vi "Teleop.vi"(10 "Match Info":T1={"Autonomous Elapsed Seconds"=0.0, "TeleOp Elapsed Seconds"=0.0, "Disabled Elapsed Seconds"=0.0, "Visited Autonomous"=FALSE, "Visited TeleOp"=FALSE, "Visited Disabled"=FALSE, "Autonomous Settings"={"Autonomous Style"=enum."Independent", "VI Refnum"=refnum}}, 11 "Call Context":T2) -> ()   [LabVIEW 2018]
doc: "This VI is called for each enabled TeleOp packet received from the DS. It is typically used to read from joysticks and other inputs and update I/O or setpoints for timed control loops. It should complete and return within 20 milliseconds or risk missing DS packets."
uses:
  <vilib>/Rock Robotics/WPI/DriverStation/WPI_DriverStationDerivedRobotMode.ctl
  <vilib>/Rock Robotics/WPI/DriverStation/WPI_DriverStationMatch Info.ctl
  <vilib>/Rock Robotics/WPI/Solenoid/WPI_SolenoidValue.ctl
  Framework/Robot Global Data.vi
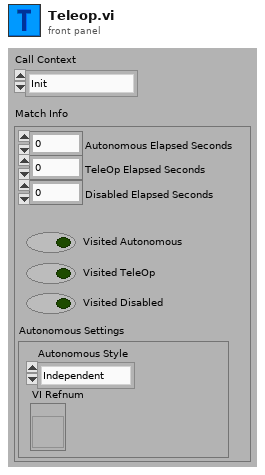
[diagram p1: front panel]
types:
  T1 = typedef "WPI_DriverStationMatch Info.ctl" = cluster{"Autonomous Elapsed Seconds":dbl, "TeleOp Elapsed Seconds":dbl, "Disabled Elapsed Seconds":dbl, "Visited Autonomous":bool, "Visited TeleOp":bool, "Visited Disabled":bool, "Autonomous Settings":cluster{"Autonomous Style":enum16{"Iterative", "Independent"}, "VI Refnum":refnum<vi>}}
  T2 = typedef "WPI_DriverStationDerivedRobotMode.ctl" = enum16{"Init", "Execute", "Stop"}
  T3 = typedef "Command Status Info.ctl" = cluster{"Name":string, "Status":T4, "notifier out":T5}
  T4 = typedef "Completion Status.ctl" = enum16{"Successful", "Aborted", "Incomplete"}
  T5 = typedef "Completion Notifier.ctl" = refnum<notifier>
  T6 = typedef "WPI_SolenoidValue.ctl" = enum16{"Off", "On", "Forward", "Reverse"}
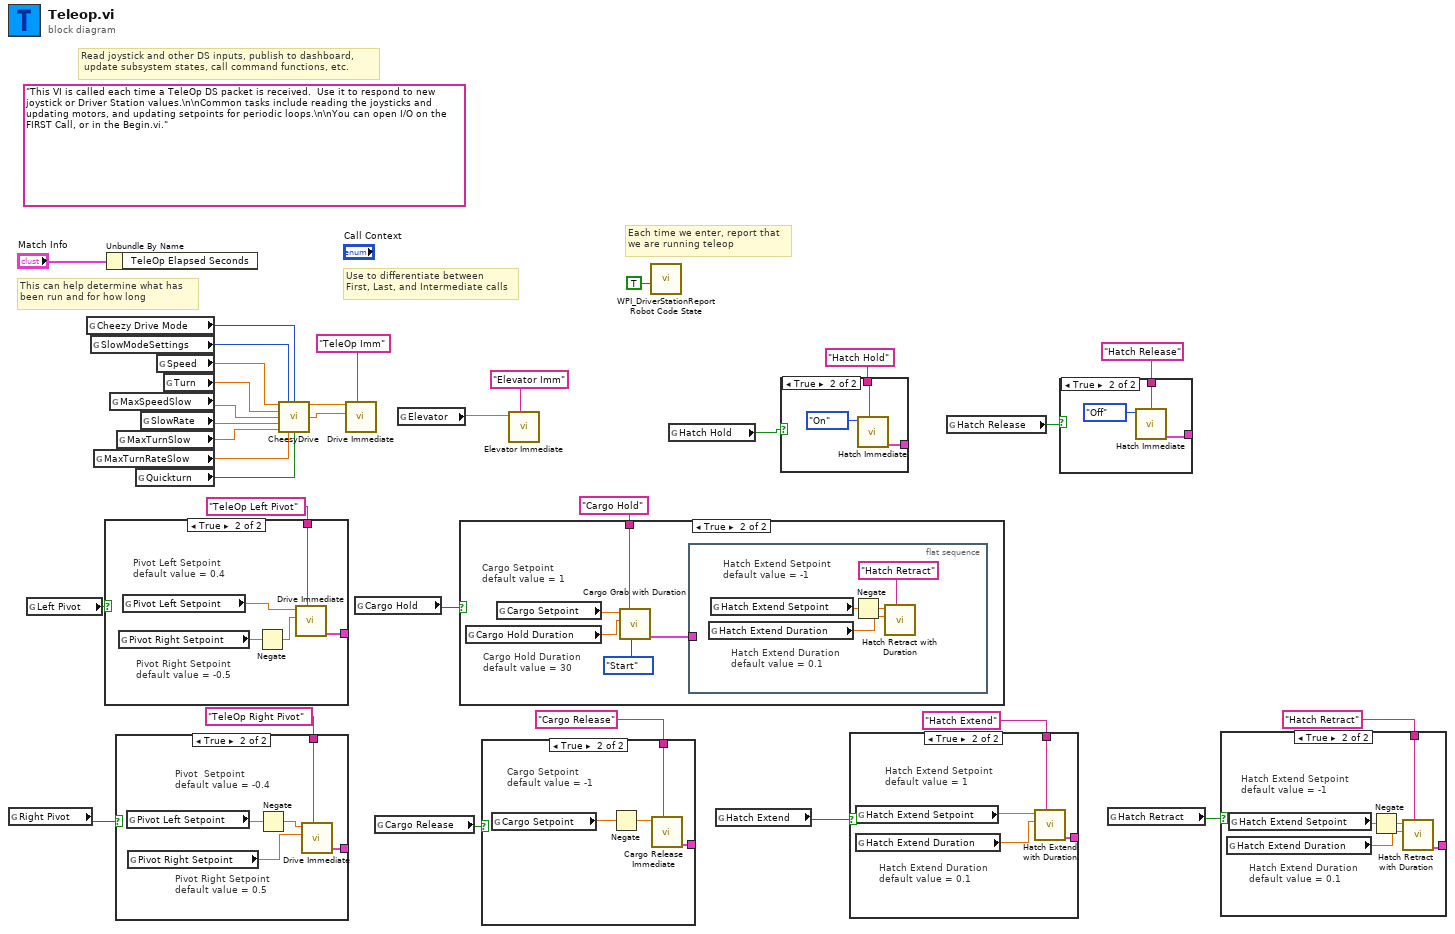
[diagram p0: block diagram]
diagram:
  (unwired) "This VI is called each time a TeleOp DS packet is received.  Use it to respond to new joystick or Driver Station values.\n\nCommon tasks include reading the joysticks and updating motors, and updating setpoints for periodic loops.\n\nYou can open I/O on the FIRST Call, or in the Begin.vi."
  # "Read joystick and other DS inputs, publish to dashboard,\n update subsystem states, call command functions, etc."
  # "Each time we enter, report that\nwe are running teleop"
  # "Use to differentiate between\nFirst, Last, and Intermediate calls"
  # "This can help determine what has\nbeen run and for how long"
  n1 = global read "Robot Global Data.vi" "Right Pivot"() -> (w27:bool)
  n2 = global read "Robot Global Data.vi" "Left Pivot"() -> (w26:bool)
  n3 = global read "Robot Global Data.vi" "Cheezy Drive Mode"() -> (w25:u32)
  n4 = global read "Robot Global Data.vi" "SlowModeSettings"() -> (w15:i32)
  n5 = global read "Robot Global Data.vi" "MaxTurnRateSlow"() -> (w17:dbl)
  n6 = case shown="True" w26 {
    tunnel: [_ w37] -> _
    tunnel: "TeleOp Left Pivot" ("Description") -> [_ w36]
    frame False {
    }
    frame True {
      # "Pivot Right Setpoint\ndefault value = -0.5"
      # "Pivot Left Setpoint\ndefault value = 0.4"
      n7 = global read "Robot Global Data.vi" "Pivot Right Setpoint"() -> (w34:dbl)
      n8 = global read "Robot Global Data.vi" "Pivot Left Setpoint"() -> (w35:dbl)
      n9 = Negate(x=w34) -> (-x=w33:dbl)
      n10 = call "Drive Immediate.vi"("Description"=w36, "Right Setpoint"=w33, "Left Setpoint"=w35) -> ("Command Info Out"=w37:T3)  [unwired: 8 in]
    }
  }
  n11 = Unbundle By Name("Match Info") -> ()  [unwired: 1 out]
  n12 = global read "Robot Global Data.vi" "MaxSpeedSlow"() -> (w20:dbl)
  n13 = case shown="True" w27 {
    tunnel: [_ w42] -> _
    tunnel: "TeleOp Right Pivot" ("Description") -> [_ w41]
    frame False {
    }
    frame True {
      # "Pivot Right Setpoint\ndefault value = 0.5"
      # "Pivot  Setpoint\ndefault value = -0.4"
      n14 = global read "Robot Global Data.vi" "Pivot Left Setpoint"() -> (w39:dbl)
      n15 = global read "Robot Global Data.vi" "Pivot Right Setpoint"() -> (w40:dbl)
      n16 = Negate(x=w39) -> (-x=w38:dbl)
      n17 = call "Drive Immediate.vi"("Description"=w41, "Right Setpoint"=w40, "Left Setpoint"=w38) -> ("Command Info Out"=w42:T3)  [unwired: 8 in]
    }
  }
  n18 = global read "Robot Global Data.vi" "MaxTurnSlow"() -> (w18:dbl)
  n19 = global read "Robot Global Data.vi" "Quickturn"() -> (w16:bool)
  n20 = global read "Robot Global Data.vi" "SlowRate"() -> (w19:dbl)
  n21 = global read "Robot Global Data.vi" "Speed"() -> (w22:dbl)
  n22 = global read "Robot Global Data.vi" "Turn"() -> (w21:dbl)
  n23 = call "CheesyDrive.vi"("Throttle"=w22, "SlowModeSettings"=w15, "SlowMode"=w25, "Wheel"=w21, "MaxSpeedSlow"=w20, "SlowRate"=w19, "MaxTurnSlow"=w18, "MaxTurnRateSlow"=w17, "Quickturn"=w16) -> ("Left PWM"=w24:dbl, "Right PWM"=w23:dbl)  [unwired: 5 in]
  n24 = call "Drive Immediate.vi"("Description"="TeleOp Imm", "Right Setpoint"=w23, "Left Setpoint"=w24) -> ()  [unwired: 8 in, 1 out]
  n25 = global read "Robot Global Data.vi" "Cargo Hold"() -> (w10:bool)
  n26 = global read "Robot Global Data.vi" "Cargo Release"() -> (w9:bool)
  n27 = global read "Robot Global Data.vi" "Elevator"() -> (w14:dbl)
  n28 = case shown="True" w10 {
    tunnel: "Cargo Hold" ("Description") -> [_ w47]
    frame False {
    }
    frame True {
      # "Cargo Hold Duration\ndefault value = 30"
      # "Cargo Setpoint\ndefault value = 1"
      n29 = global read "Robot Global Data.vi" "Cargo Hold Duration"() -> (w44:dbl)
      n30 = global read "Robot Global Data.vi" "Cargo Setpoint"() -> (w46:dbl)
      n31 = call "Cargo Grab with Duration.vi"("Synchronization"=enum16{"Start", "Wait"}."Start", "Description"=w47, "Duration (s)"=w44, "Setpoint"=w46) -> ("Command Info Out"=w43:T3)  [unwired: 7 in]
      n32 = flat-sequence {
        tunnel: w43 -> [_]
        frame #0 {
          # "Hatch Extend Setpoint\ndefault value = -1"
          # "Hatch Extend Duration\ndefault value = 0.1"
          n33 = global read "Robot Global Data.vi" "Hatch Extend Duration"() -> (w50:dbl)
          n34 = global read "Robot Global Data.vi" "Hatch Extend Setpoint"() -> (w49:dbl)
          n35 = Negate(x=w49) -> (-x=w51:dbl)
          n36 = call "Hatch Retract with Duration.vi"("Description"="Hatch Retract", "Duration (s)"=w50, "Setpoint"=w51) -> ()  [unwired: 8 in, 1 out]
        }
      }
    }
  }
  n37 = case shown="True" w9 {
    tunnel: [_ w55] -> _
    tunnel: "Cargo Release" ("Description") -> [_ w54]
    frame False {
    }
    frame True {
      # "Cargo Setpoint\ndefault value = -1"
      n38 = global read "Robot Global Data.vi" "Cargo Setpoint"() -> (w53:dbl)
      n39 = Negate(x=w53) -> (-x=w52:dbl)
      n40 = call "Cargo Release Immediate.vi"("Description"=w54, "Setpoint"=w52) -> ("Command Info Out"=w55:T3)  [unwired: 9 in]
    }
  }
  n41 = call "Elevator Immediate.vi"("Description"="Elevator Imm", "Setpoint"=w14) -> ()  [unwired: 9 in, 1 out]
  n42 = call <vilib>:"WPI_DriverStationReport Robot Code State.vi"("TeleOp"=TRUE ("Autonomous")) -> ()  [unwired: 10 in, 1 out]
  n43 = global read "Robot Global Data.vi" "Hatch Hold"() -> (w5:bool)
  n44 = global read "Robot Global Data.vi" "Hatch Extend"() -> (w4:bool)
  n45 = case shown="True" w5 {
    tunnel: "Hatch Hold" ("Description") -> [_ w58]
    tunnel: [_ w57] -> _
    frame False {
    }
    frame True {
      n46 = call "Hatch Immediate.vi"("Description"=w58, "Relay Value"=WPI_SolenoidValue."On" ("Hatch Action")) -> ("Command Info Out"=w57:T3)  [unwired: 9 in]
    }
  }
  n47 = case shown="True" w4 {
    tunnel: [_ w62] -> _
    tunnel: "Hatch Extend" ("Description") -> [_ w61]
    frame False {
    }
    frame True {
      # "Hatch Extend Duration\ndefault value = 0.1"
      # "Hatch Extend Setpoint\ndefault value = 1"
      n48 = global read "Robot Global Data.vi" "Hatch Extend Setpoint"() -> (w60:dbl)
      n49 = global read "Robot Global Data.vi" "Hatch Extend Duration"() -> (w59:dbl)
      n50 = call "Hatch Extend with Duration.vi"("Description"=w61, "Duration (s)"=w59, "Setpoint"=w60) -> ("Command Info Out"=w62:T3)  [unwired: 8 in]
    }
  }
  n51 = global read "Robot Global Data.vi" "Hatch Release"() -> (w6:bool)
  n52 = case shown="True" w6 {
    tunnel: "Hatch Release" ("Description") -> [_ w65]
    tunnel: [_ w64] -> _
    frame False {
    }
    frame True {
      n53 = call "Hatch Immediate.vi"("Description"=w65, "Relay Value"=WPI_SolenoidValue."Off" ("Hatch Action")) -> ("Command Info Out"=w64:T3)  [unwired: 9 in]
    }
  }
  n54 = global read "Robot Global Data.vi" "Hatch Retract"() -> (w3:bool)
  n55 = case shown="True" w3 {
    tunnel: [_ w70] -> _
    tunnel: "Hatch Retract" ("Description") -> [_ w69]
    frame False {
    }
    frame True {
      # "Hatch Extend Setpoint\ndefault value = -1"
      # "Hatch Extend Duration\ndefault value = 0.1"
      n56 = global read "Robot Global Data.vi" "Hatch Extend Duration"() -> (w67:dbl)
      n57 = global read "Robot Global Data.vi" "Hatch Extend Setpoint"() -> (w68:dbl)
      n58 = Negate(x=w68) -> (-x=w66:dbl)
      n59 = call "Hatch Retract with Duration.vi"("Description"=w69, "Duration (s)"=w67, "Setpoint"=w66) -> ("Command Info Out"=w70:T3)  [unwired: 8 in]
    }
  }
